vi "Read Server RPC Methods.vi"(8 "error in (no error)":errorcluster, 11 "SignalGeneratorService in":refnum<class "NiDAQmx.lvclass">) -> (0 "error out":errorcluster, 2 "Server RPC Methods":T1, 3 "SignalGeneratorService out":refnum<class "NiDAQmx.lvclass">)   [LabVIEW 2021, in "NI DAQmx_server.lvlib" / "NiDAQmx.lvclass"]
uses:
  NiDAQmx.lvclass
  typeDefs/Server gRPC UEs.ctl
  <vilib>/gRPC/LabVIEW gRPC Library/Server API/typeDefs/gRPCId Cluster.ctl
  <vilib>/gRPC/LabVIEW gRPC Library/Shared/grpcId.ctl
  NiDAQmx.lvclass/NiDAQmx.ctl
  <vilib>/gRPC/LabVIEW gRPC Library/grpc-lvsupport-release.lvlib
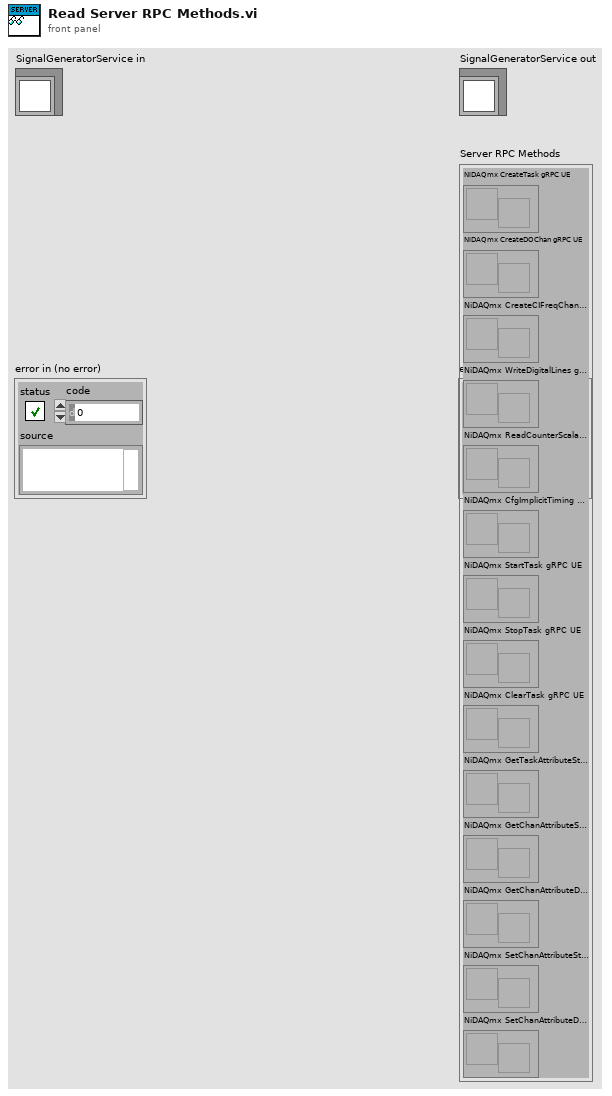
[diagram p1: front panel]
types:
  T1 = typedef "NI DAQmx_server.lvlib/NiDAQmx.lvclass/Server gRPC UEs.ctl" = cluster{"NiDAQmx CreateTask gRPC UE":refnum<user-event>, "NiDAQmx CreateDOChan gRPC UE":refnum<user-event>, "NiDAQmx CreateCIFreqChan gRPC UE":refnum<user-event>, "NiDAQmx WriteDigitalLines gRPC UE":refnum<user-event>, "NiDAQmx ReadCounterScalarF64 gRPC UE":refnum<user-event>, "NiDAQmx CfgImplicitTiming gRPC UE":refnum<user-event>, "NiDAQmx StartTask gRPC UE":refnum<user-event>, "NiDAQmx StopTask gRPC UE":refnum<user-event>, "NiDAQmx ClearTask gRPC UE":refnum<user-event>, "NiDAQmx GetTaskAttributeString gRPC UE":refnum<user-event>, "NiDAQmx GetChanAttributeString gRPC UE":refnum<user-event>, "NiDAQmx GetChanAttributeDouble gRPC UE":refnum<user-event>, "NiDAQmx SetChanAttributeString gRPC UE":refnum<user-event>, "NiDAQmx SetChanAttributeDouble gRPC UE":refnum<user-event>}
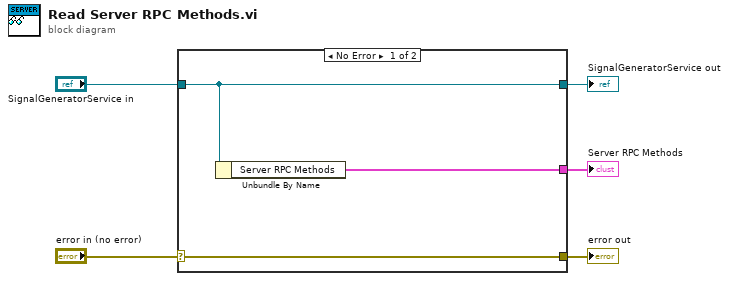
[diagram p0: block diagram]
diagram:
  n1 = case shown="No Error" "error in (no error)" {
    selector: "error in (no error)" -> [w8 w9]
    tunnel: [w8 w9] -> w4
    tunnel: [w7 w10] -> w2
    tunnel: "SignalGeneratorService in" -> [w7 w10]
    tunnel: [w6 _] -> w1
    frame No Error {
      n2 = Unbundle By Name(w7) -> ("Server RPC Methods"=w6:T1)
    }
    frame Error {
    }
  }
  "error out" <- w4
  "SignalGeneratorService out" <- w2
  "Server RPC Methods" <- w1
